vi "Configure BMI160 (C).vi"(0 "VISA resource name in":refnum<visa-resource-name>, 1 "Accel. range (g)":u8(ring) items=["+/- 2", "+/- 4", "+/- 8", "+/- 16"], 2 "Accel. rate (Hz)":u8(ring)=1 items=["3.125", "6.25", "12.5", "25", "50", "100", "200", "400", "800", "1600"], 3 "Gyro. range (dps)":u8(ring) items=["+/- 125", "+/- 250", "+/- 500", "+/- 1000", "+/- 2000"], 4 "Gyro. rate (Hz)":u8(ring) items=["6.25", "12.5", "25", "50", "100", "200", "400", "800", "1600", "3200"], 5 "Error In":errorcluster) -> (14 "VISA resource name out":refnum<visa-resource-name>, 17 "ACK ok":bool, 19 "Error out":errorcluster)   [LabVIEW 2020]
uses:
  Ctls/Cmd str.ctl
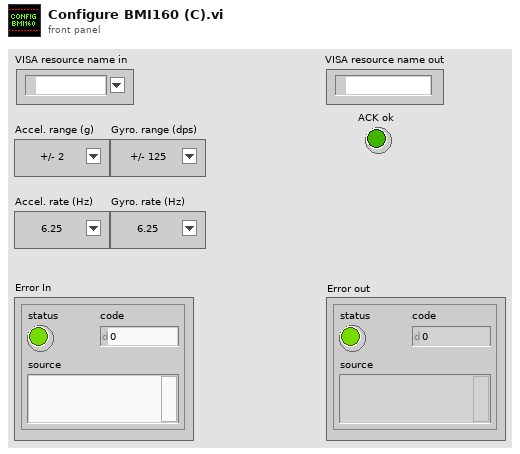
[diagram p1: front panel]
types:
  T1 = typedef "Cmd str.ctl" = string
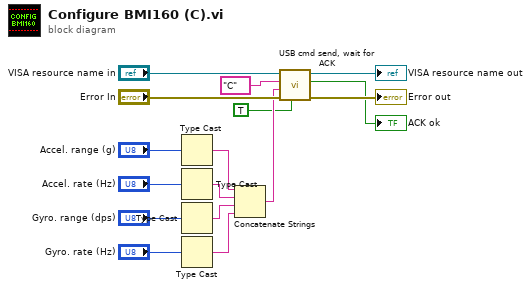
[diagram p0: block diagram]
diagram:
  n1 = Type Cast(x="Accel. range (g)") -> (*(type *) &x=w8:string)  [unwired: 1 in]
  n2 = Type Cast(x="Accel. rate (Hz)") -> (*(type *) &x=w7:string)  [unwired: 1 in]
  n3 = Type Cast(x="Gyro. range (dps)") -> (*(type *) &x=w6:string)  [unwired: 1 in]
  n4 = Type Cast(x="Gyro. rate (Hz)") -> (*(type *) &x=w5:string)  [unwired: 1 in]
  n5 = Concatenate Strings(w8, w7, w6, w5) -> (w4:string)
  n6 = call "USB cmd send, wait for ACK.vi"("Wait for ACK?"=TRUE, "Error In"="Error In", "4 byte config str"=w4, "Cmd"=T1 "C", "VISA resource name in"="VISA resource name in") -> ("Error out"=→"Error out":errorcluster, "ACK ok"=→"ACK ok":bool, "VISA resource name out"=→"VISA resource name out":refnum<visa-resource-name>)  [unwired: 1 in, 1 out]
